vi "Execution Result Color.vi"(1 "Result":T1) -> (0 "Color":string)   [LabVIEW 2015, in "HtmlReportPlugin.lvclass"]
uses:
  HtmlReportPlugin.lvclass
  Core/Execution/EXECUTION_RESULT_TYPEDEF.ctl
  Core/Execution.lvclass
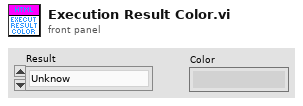
[diagram p1: front panel]
types:
  T1 = typedef "Execution.lvclass/EXECUTION_RESULT_TYPEDEF.ctl" = enum16{"Unknow", "Terminated", "Passed", "Failed", "Error"}
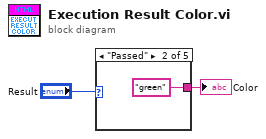
[diagram p0: block diagram]
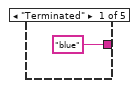
[diagram p2: hidden frame]
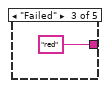
[diagram p3: hidden frame]
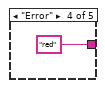
[diagram p4: hidden frame]
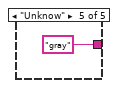
[diagram p5: hidden frame]
diagram:
  n1 = case shown="\"Passed\"" "Result" {
    tunnel: ["blue" "green" "red" "red" "gray"] -> w2
    frame "Terminated" {
    }
    frame "Passed" {
    }
    frame "Failed" {
    }
    frame "Error" {
    }
    frame "Unknow" {
    }
  }
  "Color" <- w2
